vi "Disable&Enable Controls.vi"(7 "State":T1(ring), 8 "error in (no error)":errorcluster, 11 "Controls":refnum<vi>[](array[refnum])) -> (0 "error out":errorcluster)   [LabVIEW 2010, in "CAN Log Transfer and Convert.lvlib"]
uses:
  CAN Log Transfer and Convert.lvlib
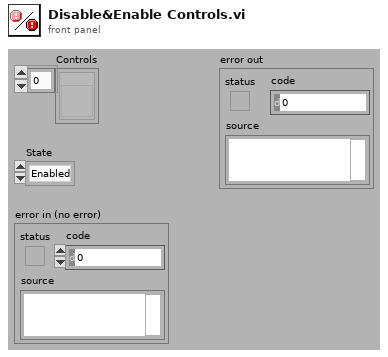
[diagram p1: front panel]
types:
  T1 = enum8{"Enabled", "Disabled", "Disabled and Grayed Out"}
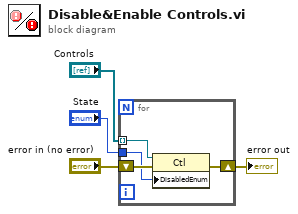
[diagram p0: block diagram]
diagram:
  n1 = for {
    tunnel: "Controls" -> [w8] mode=indexing
    shift-right: [w6] -> w3
    shift-left: "error in (no error)" -> [w7]
    tunnel: "State" -> [w5]
    n2 = property class="Ctl"(reference=w8, error in=w7, "DisabledEnum"=w5) -> (error out=w6:errorcluster)  [unwired: 1 out]
  }
  "error out" <- w3
